vi "GetStagePositionDll.vi"(8 "error in":errorcluster, 9 "Stage":T1, 11 "DevRefIn":u32) -> (0 "error out":errorcluster, 2 "Stage Position":string, 3 "DevRefOut":u32)   [LabVIEW 2020]
uses:
  StageSelector--Enum.ctl
  gclib32.lvlib
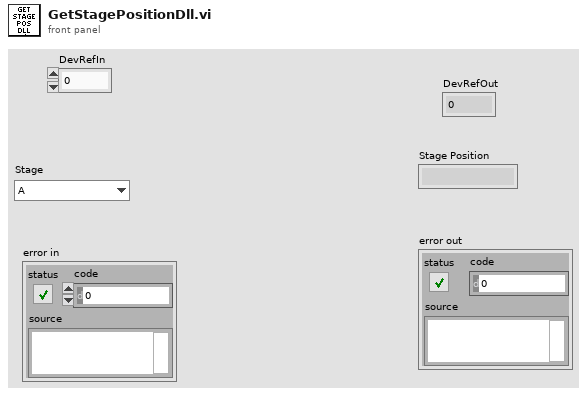
[diagram p1: front panel]
types:
  T1 = typedef "StageSelector--Enum.ctl" = enum16{"A", "B", "C", "D"}
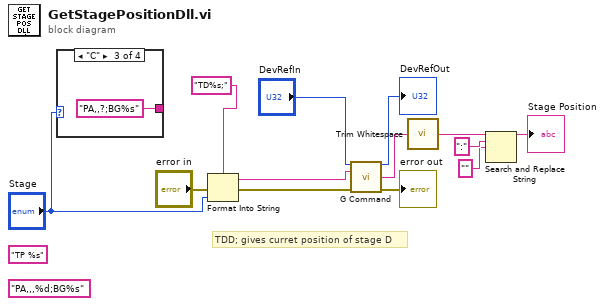
[diagram p0: block diagram]
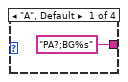
[diagram p2: hidden frame]
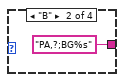
[diagram p3: hidden frame]
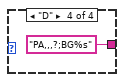
[diagram p4: hidden frame]
diagram:
  (unwired) "TP %s" ("format string")
  (unwired) "PA,,,%d;BG%s" ("format string")
  # "TDD; gives curret position of stage D"
  n1 = case shown="\"C\"" "Stage" {
    tunnel: ["PA?;BG%s" ("format string") "PA,?;BG%s" ("format string") "PA,,?;BG%s" ("format string") "PA,,,?;BG%s" ("format string")] -> _
    frame "A", Default {
    }
    frame "B" {
    }
    frame "C" {
    }
    frame "D" {
    }
  }
  n2 = Format Into String(format string="TD%s;", error in="error in", "Stage") -> (resulting string=w4:string, error out=w5:errorcluster)  [unwired: 1 in]
  n3 = call "G Command.vi"("g"="DevRefIn", "command"=w4, "error in (no error)"=w5) -> ("g out"=→"DevRefOut":u32, "buffer out"=w2:string, "error out"=→"error out":errorcluster)  [unwired: 10 in]
  n4 = call "Trim Whitespace.vi"("string"=w2) -> ("trimmed string"=w12:string)  [unwired: 1 in]
  n5 = Search and Replace String(input string=w12, search string=":", replace string="" ("replace string (\"\")")) -> (result string=→"Stage Position":string)  [unwired: 5 in, 3 out]
